vi "FromRepo.vi"(8 "error in":errorcluster, 9 "from repo cluster":T2, 10 "repository in":refnum<class "NISE_CEF_Repository.lvclass">, 11 "Systems in":refnum<class "Systems.lvclass">) -> (0 "error out":errorcluster, 2 "repository out":refnum<class "NISE_CEF_Repository.lvclass">, 3 "node":T1)   [LabVIEW 2013, in "PL Framework Configuration Tool.lvlib" / "Systems.lvclass"]
doc: "Grabs information from the Repo and stores it in the nodes."
uses:
  Systems.lvclass
  <vilib>/CEF_TreeControl/Repository/NISE_CEF_Repository.lvclass
  <vilib>/CEF_TreeControl/Node/FromRepoCluster.ctl
  <vilib>/CEF_TreeControl/Node/NodeRef.ctl
  <vilib>/CEF_TreeControl/Node/NISE_CEF_Node.lvclass
  SystemConfigRepo/SystemConfigRepo.lvclass
  SystemConfigRepo/SystemConfigRepo.lvclass/SystemConfigRepo.ctl
  Systems.lvclass/Systems.ctl
  TBM Configuration Node/TBM Configuration Node.lvclass
  Framework Configuration Classes/target configuration/PL_Target Configuration.lvclass
  <vilib>/NI/Tag Bus Module Framework/root configuration/TBM configuration.lvclass/TBM configuration.ctl
  Framework Configuration Classes/class cache/class type.ctl
  <vilib>/NI/Tag Bus Module Framework/root configuration/read metadata property.vi
  <vilib>/NI/Tag Bus Module Framework/root configuration/create GUID.vi
  <vilib>/NI/Tag Bus Module Framework/root configuration/TBM configuration.lvclass
  Framework Configuration Classes/class cache/PL_class cache.lvlib
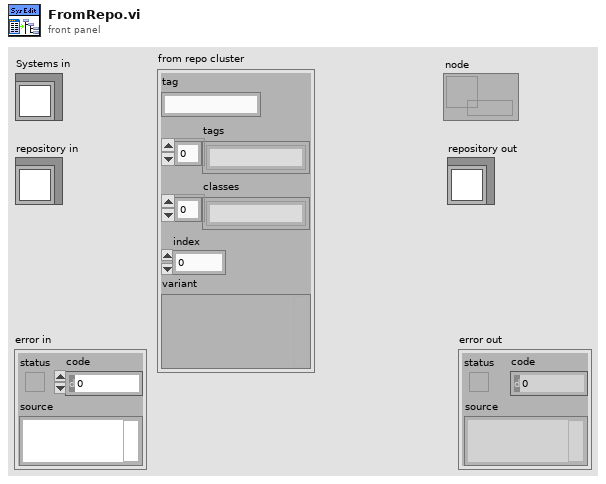
[diagram p1: front panel]
types:
  T1 = typedef "NISE_CEF_Node.lvclass/NodeRef.ctl" = refnum<data-value>
  T2 = typedef "NISE_CEF_Node.lvclass/FromRepoCluster.ctl" = cluster{"tag":string, "tags":string[], "classes":string[], "index":i32, "variant":variant}
  T3 = typedef "PLConfigurationSerializer.lvlib/targets cluster.ctl" = cluster{"Target Configuration":refnum<class "PL_Target Configuration.lvclass">, "engines":T4[]}
  T4 = typedef "PLConfigurationSerializer.lvlib/engines cluster.ctl" = cluster{"engine configuration":refnum<class "engine configuration.lvclass">, "modules":refnum<class "TBM module configuration.lvclass">[]}
  T5 = typedef "PL_class cache.lvlib/class type.ctl" = enum16{"unused", "target", "engine", "module"}
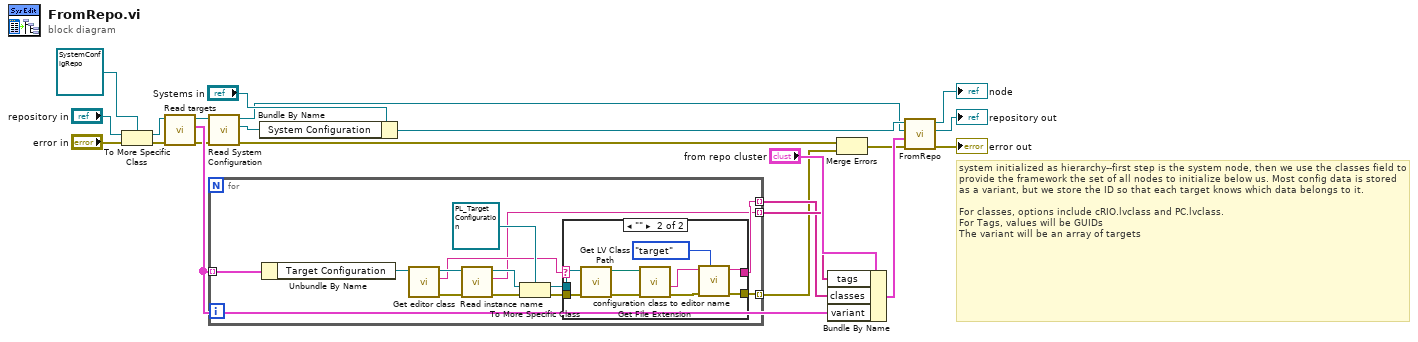
[diagram p0: block diagram]
diagram:
  # "system initialized as hierarchy--first step is the system node, then we use the classes field to provide the framework the set of all nodes to initialize below us. Most config data is stored as a variant, but we store the ID so that each target knows which data belongs to it. \n\nFor classes, options include cRIO.lvclass and PC.lvclass.\nFor Tags, values will be GUIDs\nThe variant will be an array of targets"
  n1 = To More Specific Class(target class=refnum<class "SystemConfigRepo.lvclass"> refnum ("SystemConfigRepo.lvclass"), reference="repository in", error in="error in") -> (specific class reference=w1:refnum<class "SystemConfigRepo.lvclass">, error out=w2:errorcluster)
  n2 = call "Read targets.vi"("error in"=w2, "SystemConfigRepo in"=w1) -> ("error out"=w4:errorcluster, "targets"=w8:T3[], "SystemConfigRepo out"=w5:refnum<class "SystemConfigRepo.lvclass">)  [unwired: 7 in]
  n3 = call "Read System Configuration.vi"("error in"=w4, "SystemConfigRepo in"=w5) -> ("error out"=w3:errorcluster, "System Configuration"=w7:refnum<class "PL_System Configuration.lvclass">, "SystemConfigRepo out"=w6:refnum<class "SystemConfigRepo.lvclass">)  [unwired: 7 in]
  n4 = for {
    tunnel: w8 -> [w35] mode=indexing
    tunnel: [w23] -> w12 mode=indexing
    tunnel: [w24] -> w11 mode=indexing
    tunnel: [w26] -> w9 mode=indexing
    n5 = Unbundle By Name(w35) -> ("Target Configuration"=w31:refnum<class "PL_Target Configuration.lvclass">)
    n6 = call "Get editor class.vi"("configuration in"=w31) -> ("error out"=w29:errorcluster, "editor class"=w25:string, "configuration out"=w30:refnum<class "PL_Target Configuration.lvclass">)  [unwired: 8 in]
    n7 = call <vilib>:"Read instance name.vi"("error in"=w29, "configuration in"=w30) -> ("error out"=w32:errorcluster, "instance id"=w23:string, "configuration out"=w33:refnum<class "PL_Target Configuration.lvclass">)  [unwired: 7 in]
    n8 = To More Specific Class(target class=refnum<class "PL_Target Configuration.lvclass"> refnum ("Target Configuration"), reference=w33, error in=w32) -> (specific class reference=w27:refnum<class "PL_Target Configuration.lvclass">, error out=w28:errorcluster)
    n9 = case shown="\"\"" w25 {
      selector: w25 -> [w37 _]
      tunnel: w28 -> [w36 w46]
      tunnel: w27 -> [_ w43]
      tunnel: [w36 w41] -> w26
      tunnel: [w37 w39] -> w24
      frame Default {
      }
      frame "" {
        n10 = call <vilib>:"Get LV Class Path.vi"("error in (no error)"=w46, "object"=w43) -> ("error out"=w45:errorcluster, "class path"=w44:path)  [unwired: 8 in]
        n11 = call <vilib>:"Get File Extension.vi"("error in (no error)"=w45, "file"=w44) -> ("error out"=w42:errorcluster, "filename without extension"=w40:string)  [unwired: 6 in, 2 out]
        n12 = call "configuration class to editor name.vi"("class type"=class_type."target", "error in"=w42, "configuration class name"=w40) -> ("error out"=w41:errorcluster, "editor node class name"=w39:string)  [unwired: 7 in]
      }
    }
  }
  n13 = Bundle By Name(cluster="Systems in", "System Configuration"=w7) -> (w13:refnum<class "Systems.lvclass">)
  n14 = Bundle By Name(cluster="from repo cluster", "tags"=w12, "classes"=w11, "variant"=w8) -> (w16:T2)
  n15 = Merge Errors(w3, w9) -> (w10:errorcluster)
  n16 = call-parent "FromRepo.vi"("error in"=w10, "from repo cluster"=w16, "repository in"=w6, "node in"=w13) -> ("error out"=→"error out":errorcluster, "repository out"=→"repository out":refnum<class "NISE_CEF_Repository.lvclass">, "node"=→"node":T1)  [unwired: 5 in]
